vi "Random Series Generate.vi"() -> ()   [LabVIEW 2023]
doc: "This example shows how to generate a univariate random time series with different distributions using the TSA Random Sequence Generation VI.\n\n<b>Instructions:</b>\n1) Run this VI.\n2) Select the distribution type of the random series and observe the histogram of the generated series against the ideal histogram."
uses:
  <vilib>/addons/Time Series Analysis/Utilities.llb/TSA Normal Distribution (Waveform).vi
  <vilib>/addons/Time Series Analysis/Utilities.llb/TSA Chi-Square Distribution (Waveform).vi
  <vilib>/addons/Time Series Analysis/Utilities.llb/TSA T Distribution (Waveform).vi
  <vilib>/addons/Time Series Analysis/Utilities.llb/TSA F Distribution (Waveform).vi
  <vilib>/addons/Time Series Analysis/Statistical Analysis.llb/TSA Normal Distribution Test (Waveform).vi
  <vilib>/addons/_Advanced Signal Processing/NI_AdvSigProcTSA.lvlib
panel:
  in  "stop":bool
  in  "Samples":i32=1024
  in  "Distribution Type":enum16{"Normal", "Chi-Square", "T", "F"}(ring)=enum."Chi-Square"
  out "Histogram":cluster{"Axis":dbl[], dbl[]}[](graph)
  out "Random Series":waveform(dbl)(graph)
  # "Overview: Shows how to generate a univariate random time series with different distributions using the TSA Random Sequence Generation VI.\nRequirements: LabVIEW Full Development System, Advanced Signal Processing Toolkit\nInstructions: \n1. Run this VI.\n2. Select the distribution type of the random series and observe the histogram of the generated series against the ideal histogram.\n3.  Click Stop to stop the VI."
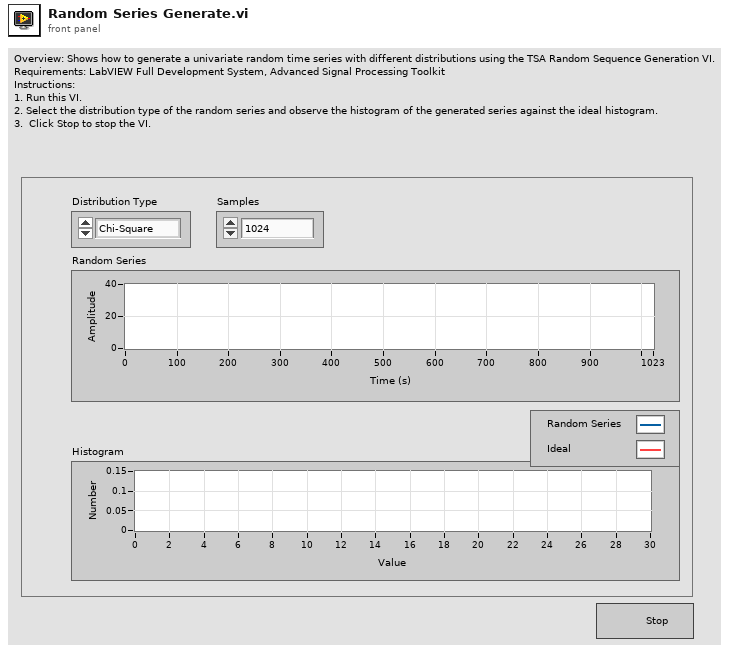
[diagram p1: front panel]
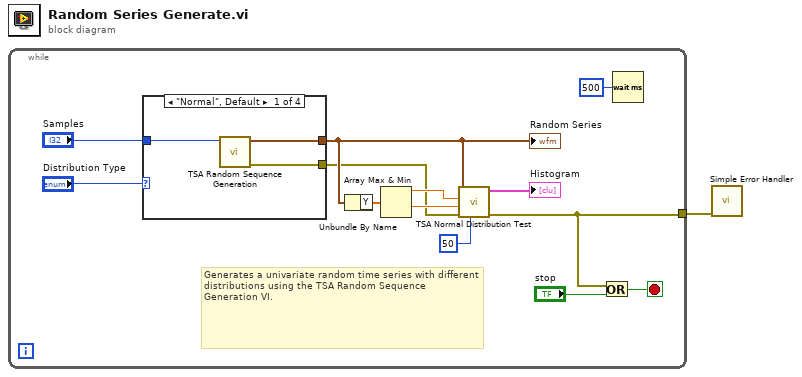
[diagram p0: block diagram]
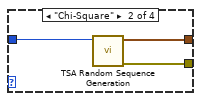
[diagram p2: hidden frame]
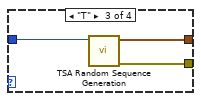
[diagram p3: hidden frame]
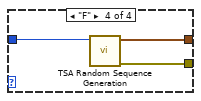
[diagram p4: hidden frame]
diagram:
  n1 = while {
    tunnel: [w2] -> w1
    stop <- w4 stop-if-true
    # "Generates a univariate random time series with different distributions using the TSA Random Sequence Generation VI."
    n2 = case shown="\"Normal\", Default" "Distribution Type" {
      tunnel: [w17 w20 w23 w26] -> w8
      tunnel: "Samples" -> [w16 w19 w22 w25]
      tunnel: [w15 w18 w21 w24] -> w3
      frame "Normal", Default {
        n3 = call-poly <vilib>:"TSA Random Sequence Generation.vi"("samples"=w16) -> ("error out"=w15:errorcluster, "Xt"=w17:waveform(dbl))  [unwired: 3 in, 6 out]
      }
      frame "Chi-Square" {
        n4 = call-poly <vilib>:"TSA Random Sequence Generation.vi"("samples"=w19) -> ("error out"=w18:errorcluster, "Xt"=w20:waveform(dbl))  [unwired: 2 in, 7 out]
      }
      frame "T" {
        n5 = call-poly <vilib>:"TSA Random Sequence Generation.vi"("samples"=w22) -> ("error out"=w21:errorcluster, "Xt"=w23:waveform(dbl))  [unwired: 2 in, 7 out]
      }
      frame "F" {
        n6 = call-poly <vilib>:"TSA Random Sequence Generation.vi"("samples"=w25) -> ("error out"=w24:errorcluster, "Xt"=w26:waveform(dbl))  [unwired: 3 in, 6 out]
      }
    }
    "Random Series" <- w8
    n7 = Unbundle By Name(w8) -> ("Y"=w7:dbl[])
    n8 = Array Max & Min(array=w7) -> (max value=w14:dbl, min value=w13:dbl)  [unwired: 2 out]
    n9 = call-poly <vilib>:"TSA Normal Distribution Test.vi"("bins"=50, "error in (no error)"=w3, "min"=w13, "max"=w14, "Xt"=w8) -> ("error out"=w2:errorcluster, "histogram"=→"Histogram":cluster{"Axis":dbl[], dbl[]}[])  [unwired: 5 out]
    n10 = Or(x=w2, y="stop") -> (x .or. y?=w4:bool)
    n11 = Wait (ms)(milliseconds to wait=u32 500 ("millisecond multiple")) -> ()  [unwired: 1 out]
  }
  n12 = call <vilib>:"Simple Error Handler.vi"("error in (no error)"=w1) -> ()  [unwired: 1 in, 8 out]
